vi "配置文件分配检索提取.vi"(11 "all rows":string[][](array[string])) -> (0 "取反信息":i32[](array[numeric]), 1 "IO配置名称索引":i32[](array[numeric]), 2 "IO配置点位地址":string[](array[string]), 3 "IO配置名称":string[](array[string]))   [LabVIEW 2017]
panel:
  out "表格控件":string[][](table)
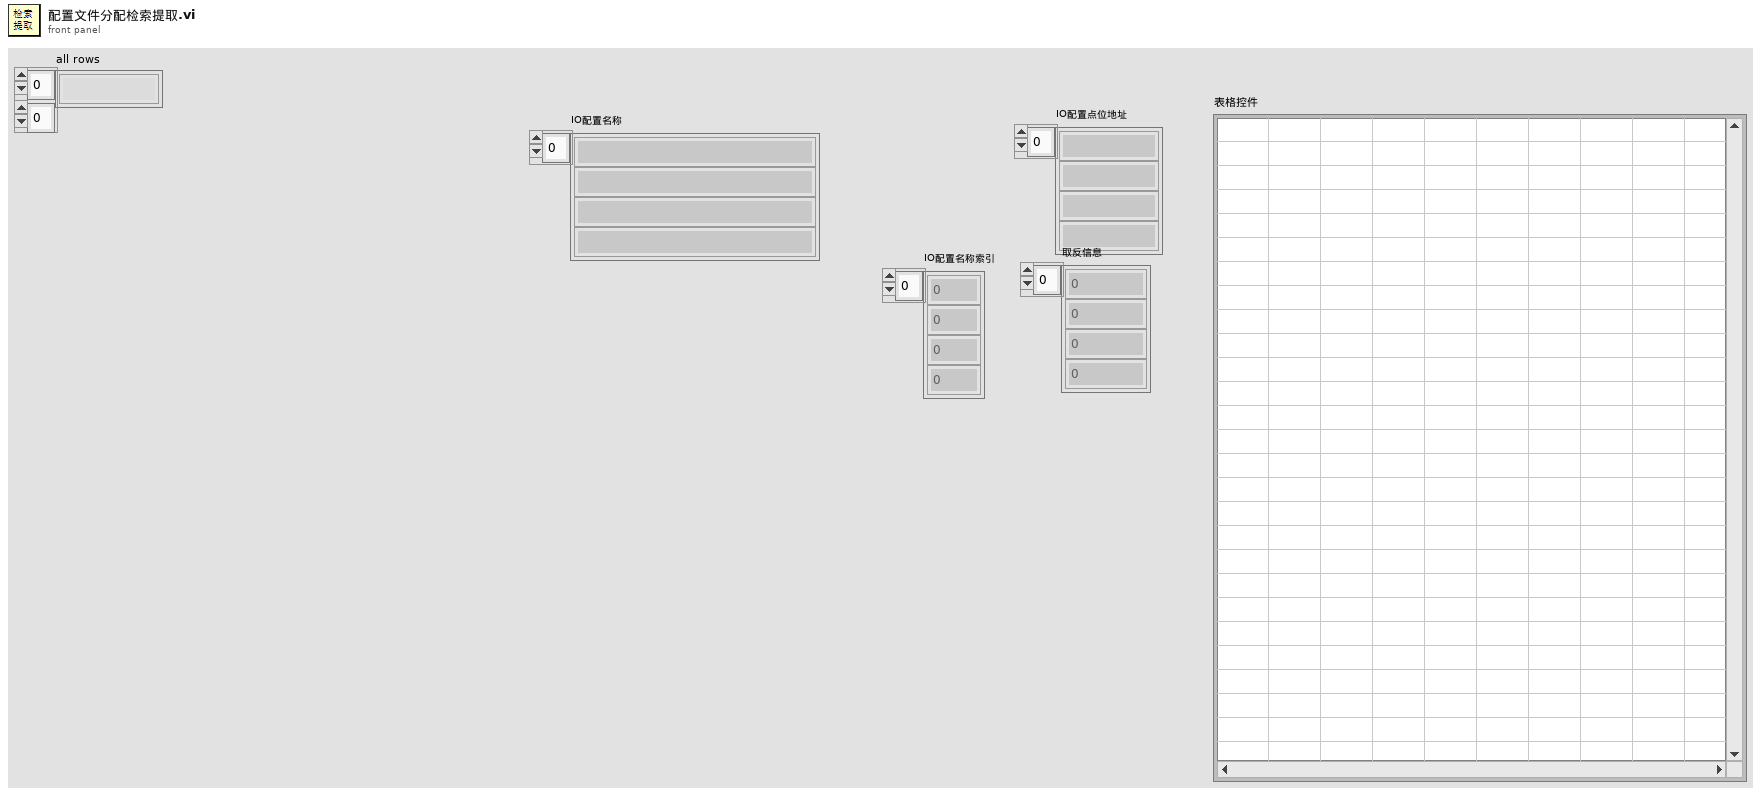
[diagram p1: front panel]
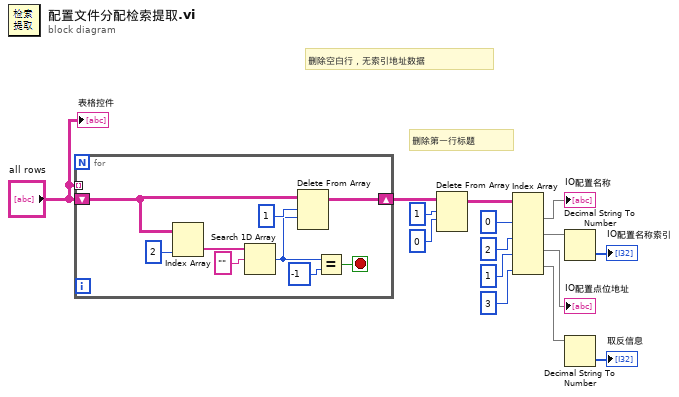
[diagram p0: block diagram]
diagram:
  # "删除空白行，无索引地址数据"
  # "删除第一行标题"
  n1 = for {
    shift-right: [w18] -> w2
    shift-left: "all rows" -> [w19]
    tunnel: "all rows" -> [_] mode=indexing
    stop <- w20 stop-if-true
    n2 = Index Array(array=w19, index (col)=2 ("禁用的索引 (列)")) -> (element=w23:string[])  [unwired: 1 in]
    n3 = Search 1D Array(1D array=w23, element="" ("元素")) -> (index of element=w16:i32)  [unwired: 1 in]
    n4 = Delete From Array(array=w19, length=1 ("长度"), index (row)=w16) -> (array with subset deleted=w18:string[][])  [unwired: 1 in, 1 out]
    n5 = Equal?(x=w16, y=-1) -> (x = y?=w20:bool)
  }
  n6 = Delete From Array(array=w2, length=1 ("长度"), index (row)=0 ("索引 (行)")) -> (array with subset deleted=w13:string[][])  [unwired: 1 in, 1 out]
  n7 = Index Array(array=w13, index (col) #1=0 ("禁用的索引 (列)"), index (col) #2=2 ("禁用的索引 (列)"), index (col) #3=1 ("禁用的索引 (列)"), index (col) #4=3 ("禁用的索引 (列)")) -> (element #1=→"IO配置名称":string[], element #2=w7:string[], element #3=→"IO配置点位地址":string[], element #4=w4:string[])  [unwired: 4 in]
  n8 = Decimal String To Number(string=w7) -> (number=→"IO配置名称索引":i32[])  [unwired: 2 in, 1 out]
  n9 = Decimal String To Number(string=w4) -> (number=→"取反信息":i32[])  [unwired: 2 in, 1 out]
  "表格控件" <- "all rows"
